vi "PicoScope2000aExampleEts.vi"() -> ()   [LabVIEW 2010]
uses:
  shared/PicoBuffers.ctl
  shared/Buffer and Transfer Settings.ctl
  shared/Acquisition Settings.ctl
  PicoScope2000aLib/PicoScope2000aAnalogChannelSettings.ctl
panel:
  in  "Write to TDMS":bool
  in  "Channel B Settings":T1={"Enabled"=FALSE, "Coupling"=1, "Range"=6, "Analogue Offset"=0.0} {"Range" items=["20 mV"=1, "50 mV"=2, "100 mV"=3, "200 mV"=4, "500 mV"=5, "1 V"=6, "2 V"=7, "5 V"=8, "10 V"=9, "20 V"=10]; "Coupling" items=["AC", "DC"]}
  in  "Trigger Settings":T2={"Trigger Enabled"=TRUE, "Trigger Source"=enum."Channel A", "Trigger Threshold (Volts)"=0.0, "Trigger Direction"=2, "Trigger Delay (samples)"=0, "Auto Trigger Time (ms)"=1000} {"Trigger Direction" items=["Rising"=2, "Falling"=3]}
  out "Device Info":T3
  in  "Channel A Settings":T1={"Enabled"=TRUE, "Coupling"=1, "Range"=6, "Analogue Offset"=0.0} {"Analogue Offset" format="%#_6p"; "Range" items=["20 mV"=1, "50 mV"=2, "100 mV"=3, "200 mV"=4, "500 mV"=5, "1 V"=6, "2 V"=7, "5 V"=8, "10 V"=9, "20 V"=10]; "Coupling" items=["AC", "DC"]}
  out "Properties Panel":T4 {"Max Total Capture Time Available (sec)" format="%.3p"; "Sample Frequency" format="%.3p"; "Sample Rate" format="%.3p"; "Max Samples Available" format="%.3p"; "Total Capture Time (sec)" format="%.3p"}
  out "EtsTimeValues":i64[](array[numeric])
  in  "etsInterleave":i16=10
  in  "etsCycles":i16=100
  in  "ETS Mode":u32(ring)=1 items=["PS2000A_ETS_OFF", "PS2000A_ETS_FAST", "PS2000A_ETS_SLOW"]
  out "overflow":i16 format="%06b"
  in  "Apply Settings":bool
  out "error out":errorcluster
  in  "Data file":path=path "PicoScope2000aExampleETS ChA Data"
  in  "Buffer and Transfer Settings":T5={"startIndex"=0, "Samples"=1000, "Down Sample Ratio"=1, "Down-Sample Mode"=0} {"Down-Sample Mode" items=["RAW none"=2147483648, "None"=0, "Aggregate"=1, "Decimate"=2, "Average"=4]; "Down Sample Ratio" step=1; "Samples" format="%_6p"}
  in  "Acquisition Settings":T6={"preTriggerSamples"=0, "postTriggerSamples"=1000, "timebase"=0} {"postTriggerSamples" format="%_6p"; "preTriggerSamples" format="%_6p"}
  in  "stop":bool
  out "Channel A":cluster{i32, sgl, "Data":dbl[]}[](graph)
  in  "Serial Number":string
  in  "Use Serial Number":bool
  in  "error in (no error)":errorcluster
  # "Bit 0 = ChA"
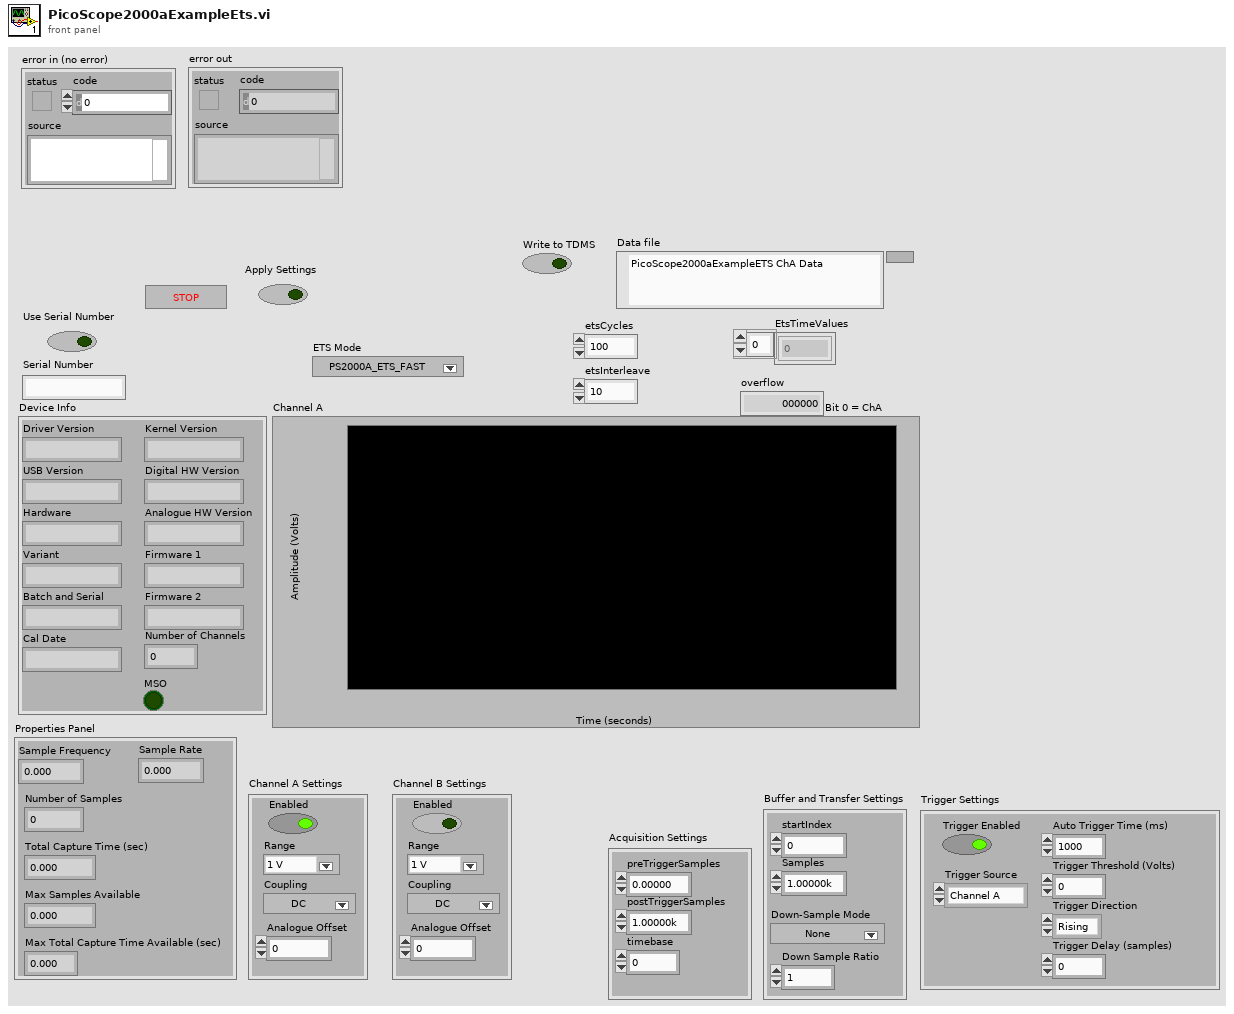
[diagram p1: front panel]
types:
  T1 = typedef "PicoScope2000aAnalogChannelSettings.ctl" = cluster{"Enabled":bool, "Coupling":i16, "Range":u32, "Analogue Offset":sgl}
  T2 = cluster{"Trigger Enabled":bool, "Trigger Source":enum16{"Channel A", "Channel B", "Channel C", "Channel D", "Ext."}, "Trigger Threshold (Volts)":dbl, "Trigger Direction":u16, "Trigger Delay (samples)":u32, "Auto Trigger Time (ms)":i16}
  T3 = cluster{"Driver Version":string, "USB Version":string, "Hardware":string, "Variant":string, "Batch and Serial":string, "Cal Date":string, "Kernel Version":string, "Digital HW Version":string, "Analogue HW Version":string, "Firmware 1":string, "Firmware 2":string, "MSO":bool, "Number of Channels":i16}
  T4 = cluster{"Sample Frequency":sgl, "Sample Rate":sgl, "Max Samples Available":i32, "Number of Samples":u32, "Total Capture Time (sec) ":sgl, "Max Total Capture Time Available (sec)":sgl}
  T5 = typedef "Buffer and Transfer Settings.ctl" = cluster{"startIndex":u64, "Samples":u64, "Down Sample Ratio":u64, "Down-Sample Mode":u32}
  T6 = typedef "Acquisition Settings.ctl" = cluster{"preTriggerSamples":u64, "postTriggerSamples":u64, "timebase":u32}
  T7 = typedef "PicoBuffers.ctl" = cluster{"Max Buffer Pointers":u64[][][], "Min Buffer Pointers":u64[][][], "StreamingDataInfo":cluster{"Channel":u32, "Down-Sample Mode":u32, "PICO_DATA_TYPE":enum32{"PICO_INT8_T", "PICO_INT16_T", "PICO_INT32_T", "PICO_UINT32_T", "PICO_INT64_T", ""}, "Samples":i32, "bufferIndex":u64, "startIndex":i32, "overflow":i16}[][]}
  T8 = enum16{"open", "open or create", "create or replace", "create", "open (read-only)"}
  T9 = cluster{"Sample Frequency":sgl, "Sample Internal":sgl, "Max Samples Available":i32, "Number of Samples":u32, "Total Capture Time (sec) ":sgl, "Max Total Capture Time Available (sec)":sgl}
  T10 = cluster{"Channel A Buffer":i16[], "Channel B Buffer":i16[], "Channel C Buffer":i16[], "Channel D Buffer":i16[], "Channel E Buffer":i16[], "Channel F Buffer":i16[], "Channel G Buffer":i16[], "Channel H Buffer":i16[], "Port 0 Buffer":i16[], "Port 1 Buffer":i16[]}[]
  T11 = cluster{"Channel A Buffer":i16[], "Channel B Buffer":i16[], "Channel C Buffer":i16[], "Channel D Buffer":i16[], "Channel E Buffer":i16[], "Channel F Buffer":i16[], "Channel G Buffer":i16[], "Channel H Buffer":i16[], "Port 0 Buffer":i16[], "Port 1 Buffer":i16[]}
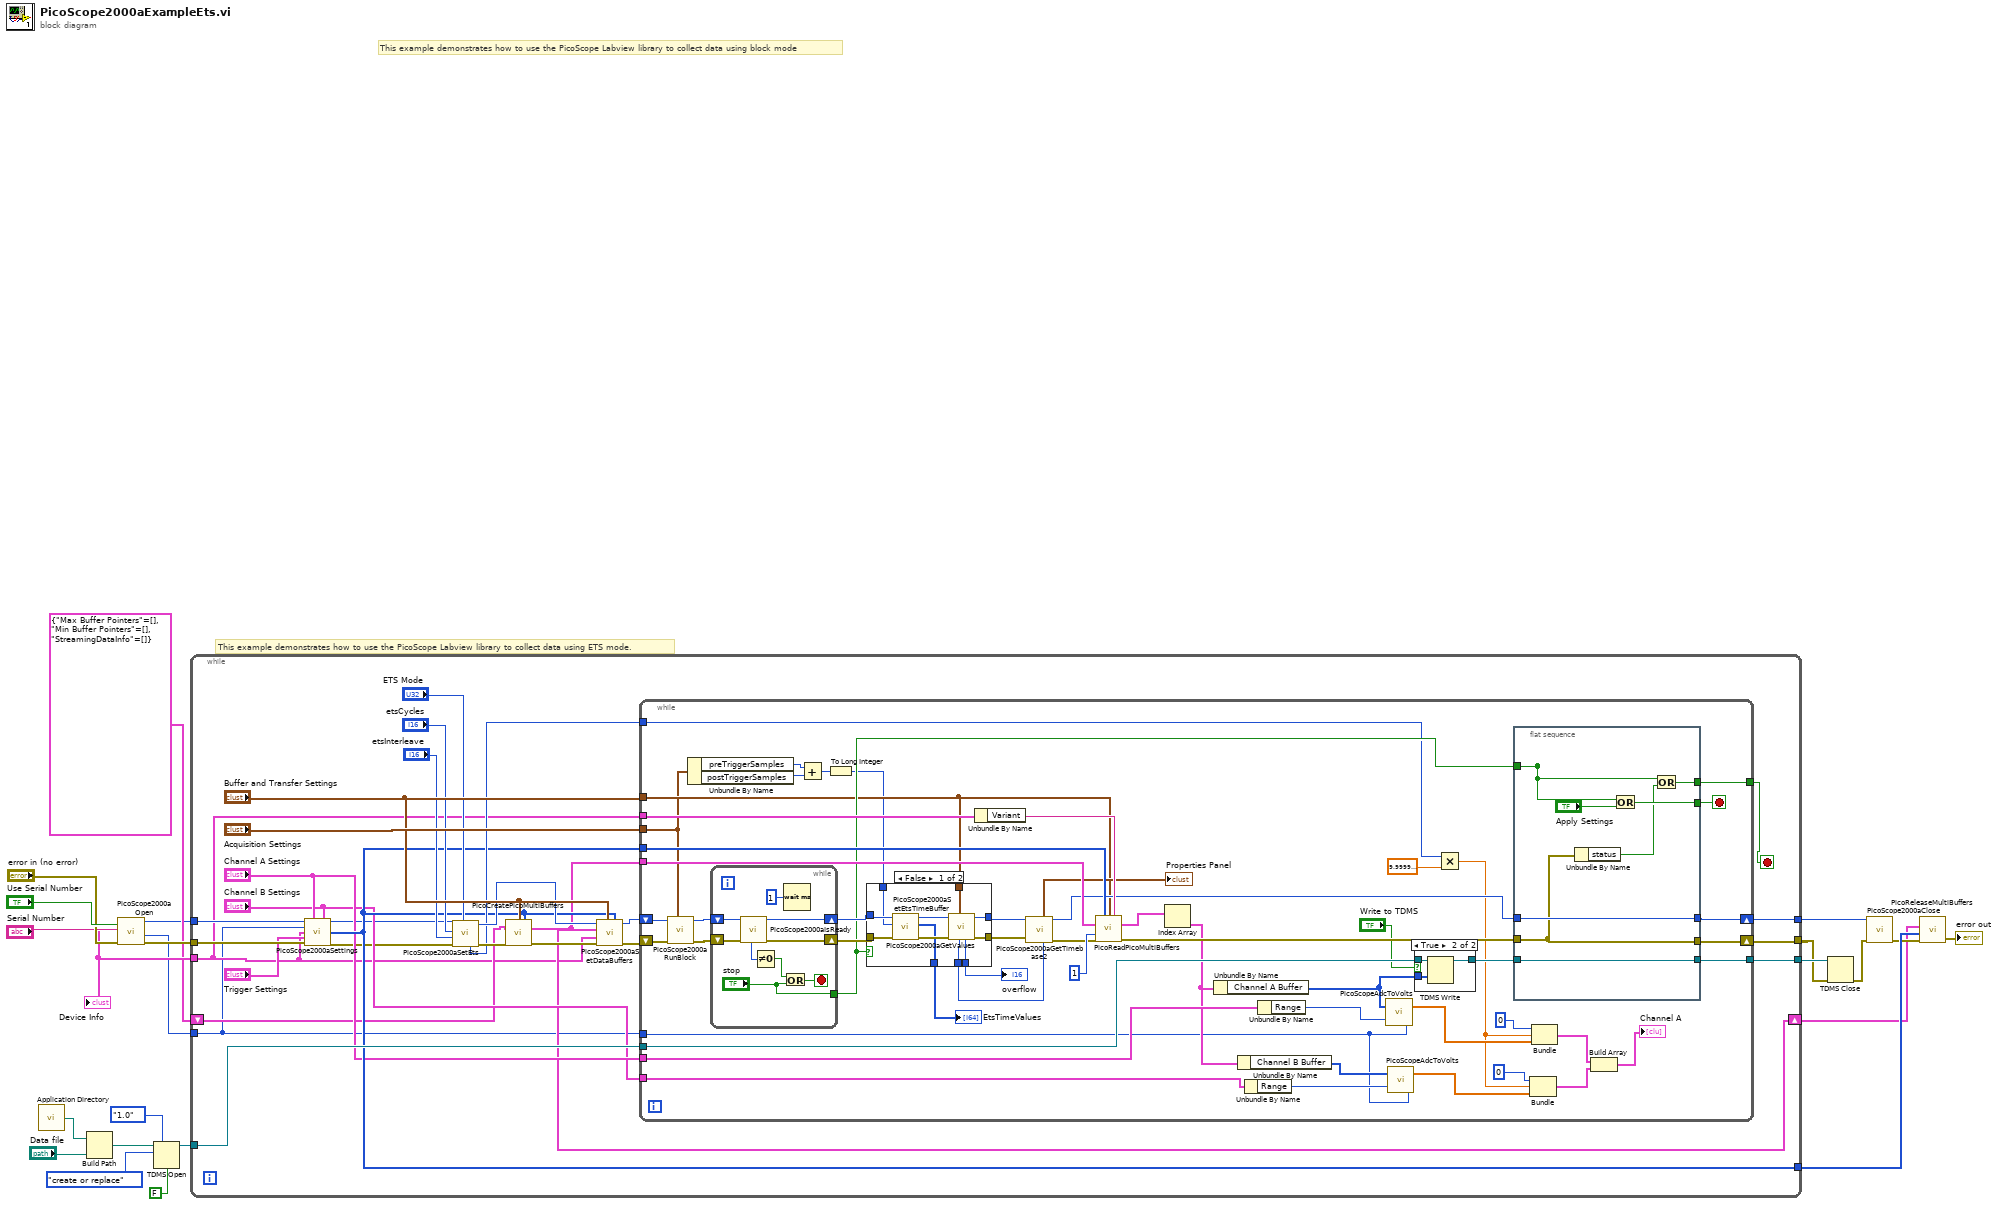
[diagram p0: block diagram]
diagram:
  # "This example demonstrates how to use the PicoScope Labview library to collect data using ETS mode."
  # "This example demonstrates how to use the PicoScope Labview library to collect data using block mode"
  n1 = call <vilib>:"Application Directory.vi"() -> ("Application Directory"=w17:path)
  n2 = Build Path(base path=w17, name or relative path="Data file") -> (appended path=w18:path)
  n3 = call "PicoScope2000aOpen.vi"("Serial Number"="Serial Number", "Use Serial Number"="Use Serial Number", "error in (no error)"="error in (no error)") -> ("error out"=w10:errorcluster, "Max Adc value"=w3:i16, "Device Info"=w9:T3, "handle"=w4:i16)  [unwired: 3 in, 2 out]
  "Device Info" <- w9
  n4 = TDMS Open(6:FALSE ("disable buffering? (T)"), 7:enum16{"1.0", "2.0"}."1.0" ("file format version (2.0)"), 10:T8."create or replace" ("operation (0:open)"), 11:w18) -> (3:w15:refnum<k34>)  [unwired: 2 in, 1 out]
  n5 = while {
    tunnel: [w35] -> w23
    tunnel: [w47] -> w16
    tunnel: w15 -> [w50]
    tunnel: w10 -> [w30]
    tunnel: [w48] -> w2
    tunnel: [w45] -> w7
    tunnel: w9 -> [w25]
    shift-right: [w31] -> w5
    shift-left: T7 {"Max Buffer Pointers"=[], "Min Buffer Pointers"=[], "StreamingDataInfo"=[]} ("Data Pointers") -> [w32]
    tunnel: w4 -> [w29]
    tunnel: w3 -> [w24]
    stop <- w46 stop-if-true
    n6 = call "PicoScope2000aSettings.vi"("handle in"=w29, "Channel A Settings"="Channel A Settings", "Channel C Settings"="Channel B Settings", "Max_adc"=w24, "Device Info"=w25, "Trigger Settings"="Trigger Settings", "error in"=w30) -> ("handle out"=w27:i16, "Enabled Array"=w35:i16[], "error out"=w28:errorcluster)  [unwired: 6 in]
    n7 = call "PicoScope2000aSetEts.vi"("ETS Mode"="ETS Mode", "error in (no error)"=w28, "etsInterleave"="etsInterleave", "etsCycles"="etsCycles", "handle in"=w27) -> ("error out"=w41:errorcluster, "handle out"=w40:i16, "sampleTimePicoseconds"=w39:i32)  [unwired: 4 in]
    n8 = call "PicoCreatePicoMultiBuffers.vi"("Buffer and Transfer Settings"="Buffer and Transfer Settings", "enabled array"=w35, "Data Pointers In"=w32, "error in (no error)"=w41) -> ("Data Pointers"=w31:T7, "error out"=w51:errorcluster)  [unwired: 10 in]
    n9 = call "PicoScope2000aSetDataBuffers.vi"("enabled array"=w35, "Buffer and Transfer Settings"="Buffer and Transfer Settings", "error in (no error)"=w51, "Device Info"=w25, "Data Pointers In"=w31, "handle in"=w40) -> ("error out"=w44:errorcluster, "handle out"=w43:i16)  [unwired: 4 in]
    n10 = while {
      tunnel: w31 -> [w105]
      tunnel: "Buffer and Transfer Settings" -> [w73]
      tunnel: w35 -> [w100]
      tunnel: "Channel A Settings" -> [w99]
      tunnel: "Acquisition Settings" -> [w68]
      tunnel: w24 -> [w57]
      tunnel: w25 -> [w97]
      tunnel: [w88] -> w46
      shift-right: [w92] -> w48
      shift-left: w44 -> [w82]
      shift-right: [w86] -> w45
      shift-left: w43 -> [w83]
      tunnel: w50 -> [w104]
      tunnel: [w90] -> w47
      tunnel: w39 -> [w71]
      tunnel: "Channel B Settings" -> [w56]
      stop <- w87 stop-if-true
      n11 = call "PicoScope2000aRunBlock.vi"("Acquisition Settings"=w68, "error in (no error)"=w82, "handle in"=w83) -> ("error out"=w102:errorcluster, "handle out"=w101:i16)  [unwired: 5 in, 2 out]
      n12 = Unbundle By Name(w68) -> ("preTriggerSamples"=w67:u64, "postTriggerSamples"=w66:u64)
      n13 = while {
        shift-right: [w138] -> w84
        shift-left: w102 -> [w139]
        shift-right: [w137] -> w85
        shift-left: w101 -> [w136]
        tunnel: ["stop"] -> w81
        stop <- w133 stop-if-true
        n14 = call "PicoScope2000aIsReady.vi"("error in (no error)"=w139, "handle in"=w136) -> ("error out"=w138:errorcluster, "handle out"=w137:i16, "ready"=w135:i16)  [unwired: 7 in]
        n15 = Not Equal To 0?(x=w135) -> (x != 0?=w134:bool)
        n16 = Or(x=w134, y="stop") -> (x .or. y?=w133:bool)
        n17 = Wait (ms)(milliseconds to wait=u32 1) -> ()  [unwired: 1 out]
      }
      n18 = Add(x=w67, y=w66) -> (x+y=w65:u64)
      n19 = To Long Integer(number=w65) -> (32bit integer=w64:i32)
      n20 = case shown="False" w81 {
        tunnel: w84 -> [w115 w121]
        tunnel: w85 -> [w112 w122]
        tunnel: [w120 w122] -> w76
        tunnel: [w119 w121] -> w77
        tunnel: w73 -> [w118 _]
        tunnel: [w117 _] -> w80
        tunnel: [w116 _] -> w79
        tunnel: [w111 _] -> w70
        tunnel: w64 -> [w110 _]
        frame False {
          n21 = call "PicoScope2000aSetEtsTimeBuffer.vi"("error in (no error)"=w115, "bufferLth"=w110, "handle in"=w112) -> ("error out"=w114:errorcluster, "EtsTimeValues"=w111:i64[], "handle out"=w113:i16)  [unwired: 6 in]
          n22 = call "PicoScope2000aGetValues.vi"("Buffer and Transfer Settings"=w118, "error in (no error)"=w114, "handle in"=w113) -> ("error out"=w119:errorcluster, "handle out"=w120:i16, "overflow"=w117:i16, "noOfSamples"=w116:u64)  [unwired: 5 in]
        }
        frame True {
        }
      }
      "overflow" <- w80
      "EtsTimeValues" <- w70
      n23 = Unbundle By Name(w97) -> ("Variant"=w98:string)
      n24 = call "PicoScope2000aGetTimebase2.vi"("Number of Samples"=w79, "error in (no error)"=w77, "handle in"=w76) -> ("error out"=w75:errorcluster, "handle out"=w74:i16, "Properties Panel"=→"Properties Panel":T9)  [unwired: 6 in]
      n25 = call "PicoReadPicoMultiBuffers.vi"("enabled array"=w100, "Buffer and Transfer Settings"=w73, "Variant"=w98, "Data Pointers"=w105, "No of Buffers"=1, "error in (no error)"=w75) -> ("MultiBuffers (Max or non-aggregated)"=w103:T10, "error out"=w89:errorcluster)  [unwired: 7 in, 1 out]
      n26 = Index Array(array=w103) -> (element=w60:T11)  [unwired: 1 in]
      n27 = Unbundle By Name(w60) -> ("Channel A Buffer"=w93:i16[])
      n28 = Unbundle By Name(w60) -> ("Channel B Buffer"=w59:i16[])
      n29 = Unbundle By Name(w56) -> ("Range"=w58:u32)
      n30 = Unbundle By Name(w99) -> ("Range"=w94:u32)
      n31 = call "PicoScopeAdcToVolts.vi"("Max_adc"=w57, "Range Index"=w94, "Data"=w93) -> ("Data"=w69:dbl[])
      n32 = call "PicoScopeAdcToVolts.vi"("Max_adc"=w57, "Range Index"=w58, "Data"=w59) -> ("Data"=w61:dbl[])
      n33 = case shown="True" "Write to TDMS" {
        tunnel: w104 -> [w106 w109]
        tunnel: w93 -> [_ w108]
        tunnel: [w106 w107] -> w91
        frame False {
        }
        frame True {
          n34 = TDMS Write(0:w109, 9:w108) -> (4:w107:refnum<k34>)  [unwired: 4 in, 3 out]
        }
      }
      n35 = Multiply(x=w71, y=sgl 1e-12) -> (x*y=w62:sgl)
      n36 = flat-sequence {
        tunnel: [w130] -> w87
        tunnel: [w123] -> _
        tunnel: [w127] -> w88
        tunnel: w74 -> [w126]
        tunnel: [w126] -> w86
        tunnel: w89 -> [w125]
        tunnel: [w125] -> w92
        tunnel: [w124] -> w90
        tunnel: w91 -> [w124]
        tunnel: w81 -> [w123]
        frame #0 {
          n37 = Unbundle By Name(w125) -> ("status"=w128:bool)
          n38 = Or(x=w123, y="Apply Settings") -> (x .or. y?=w130:bool)
          n39 = Or(x=w123, y=w128) -> (x .or. y?=w127:bool)
        }
      }
      n40 = Bundle(0, w62, "Data"=w61) -> (w55:cluster{i32, sgl, "Data":dbl[]})  [unwired: 1 in]
      n41 = Bundle(0, w62, "Data"=w69) -> (w54:cluster{i32, sgl, "Data":dbl[]})  [unwired: 1 in]
      n42 = Build Array(w54, w55) -> (→"Channel A":cluster{i32, sgl, "Data":dbl[]}[])
    }
  }
  n43 = TDMS Close(8:w2, 11:w16) -> (0:w1:errorcluster)  [unwired: 1 out]
  n44 = call "PicoScope2000aClose.vi"("error in (no error)"=w1, "handle in"=w7) -> ("error out"=w8:errorcluster)  [unwired: 8 in, 1 out]
  n45 = call "PicoReleaseMultiBuffers.vi"("error in (no error)"=w8, "Enabled array"=w23, "Data Pointers"=w5) -> ("error out"=→"error out":errorcluster)  [unwired: 7 in, 1 out]
